vi "Modbus_FSM_Polarization_Control.vi"() -> ()   [LabVIEW 2021]
uses:
  <vilib>/Plasmionique/MB Master/MB_ADU/MB_ADU.lvclass/MB_ADU.ctl
  <vilib>/Plasmionique/MB Master/MB_ADU/Read TX Data.vi
  <vilib>/Plasmionique/MB Master/MB_ADU/Read RX Data.vi
  <vilib>/Plasmionique/MB Master/MB_ADU/Read RX Timestamp.vi
  <vilib>/Plasmionique/MB Master/MB_Master_Serial/MB_Master_Serial.lvclass
  C:/Program Files/National Instruments/LabVIEW 2021/vi.lib/Plasmionique/MB Master/MB_Master/MB_Master.lvclass
  <vilib>/Plasmionique/MB Master/MB_ADU/MB_ADU.lvclass
  <vilib>/Plasmionique/MB Master/MB_Master/MB_Master.lvclass
  <vilib>/Plasmionique/MB Master/MB Master.lvlib
panel:
  out "Full Excitation Scan?":bool=TRUE
  out "Current Excitation HWP Segments":u8=230
  out "Initial Excitation QWP Segments":u8
  out "Current Excitation\nQWP angle":sgl
  in  "Event Registration Refnum":refnum<event-registration>
  in  "stop":bool
  in  "Scan Angle\nExcitation QWP":dbl=45.0
  in  "Excitation Full Scan":bool
  in  "Excitation  QWP Angle":dbl(slide)=1.0 min=0.0 max=180.0 step=0.001 scale=0.0..180.0
  out "Reset Modbus?":bool=TRUE
  in  "Modbus Address":refnum<visa-resource-name>="COM21"
  in  "Collection QWP Angle":dbl(slide)=1.0 min=0.0 max=180.0 step=0.001 scale=0.0..180.0
  in  "Scan Angle \nCollection QWP":dbl=45.0
  in  "Excitation  HWP Angle":dbl(slide)=1.0 min=0.0 max=180.0 step=0.001 scale=0.0..180.0
  in  "Scan Angle \nExcitation HWP":dbl=45.0
  in  "Collection HWP Angle":dbl(slide)=1.0 min=0.0 max=180.0 step=0.1 scale=0.0..180.0
  in  "Scan Angle\nCollection HWP":dbl=45.0
  out "Def Pos CH3":u16[](array[numeric])
  out "Def Pos CH2":u16[](array[numeric])
  out "Def Pos CH1":u16[](array[numeric])
  out "Def Pos CH0":u16[](array[numeric])
  in  "Direction Exc QWP":bool
  in  "Direction Exc HWP":bool
  in  "Direction QWP":bool
  in  "Direction HWP":bool
  out "CH1 Steps/deg":u16=400
  out "CH0 Steps/deg":u16=400
  out "Current Collection HWP Segments":u8
  out "Initial Collection HWP Segments":u8=230
  out "CH2 Steps/deg":u16=400
  out "CH3 Steps/deg":u16=400
  out "Current Collection QWP Segment":u8
  out "Initial Collection QWP Segments":u8=230
  out "Current Collection \nHWP angle":sgl
  out "Current Collection\nQWP angle":sgl
  out "Full Collection Scan?":bool=TRUE
  out "Current Excitation QWP Segments":u8
  out "Initial Excitation HWP Segments":u8=230
  out "Current Excitation\nHWP angle":sgl
  out "Def Pos CH0 Ind":bool=TRUE
  out "Def Pos CH1 Ind":bool=TRUE
  out "Def Pos CH2 Ind":bool=TRUE
  out "Def Pos CH3 Ind":bool=TRUE
  out "Power Dependence?":bool=TRUE
  out "Last RX":string
  out "Last TX":string
  out "Last RX Time":string
  out "dt (ms)":u32=4
  out "Open?":bool
  out "Last Error Time":string
  out "Last Error Status":errorcluster
  in  "Reset Motor":bool
  in  "Excitation QWP":bool
  in  "Excitation HWP":bool
  in  "Collection QWP":bool
  in  "Collection HWP":bool
  in  "Scan Collection polarization":bool
  in  "Absolute Move CH0":bool=TRUE caption="Move to Default"
  in  "Absolute Move CH1":bool=TRUE
  in  "Absolute Move CH2":bool=TRUE
  in  "Absolute Move CH3":bool=TRUE
  in  "Set CH0 Default Position":bool=TRUE caption="Set Default"
  in  "Set CH1 Default Position":bool=TRUE
  in  "Set CH2 Default Position":bool=TRUE
  in  "Set CH3 Default Position":bool=TRUE
  in  "Scan Excitation LP":bool
  in  "Scan Collection LP":bool
  # "Rotation"
  # "Scan"
  # "Direction"
  # "Rotate"
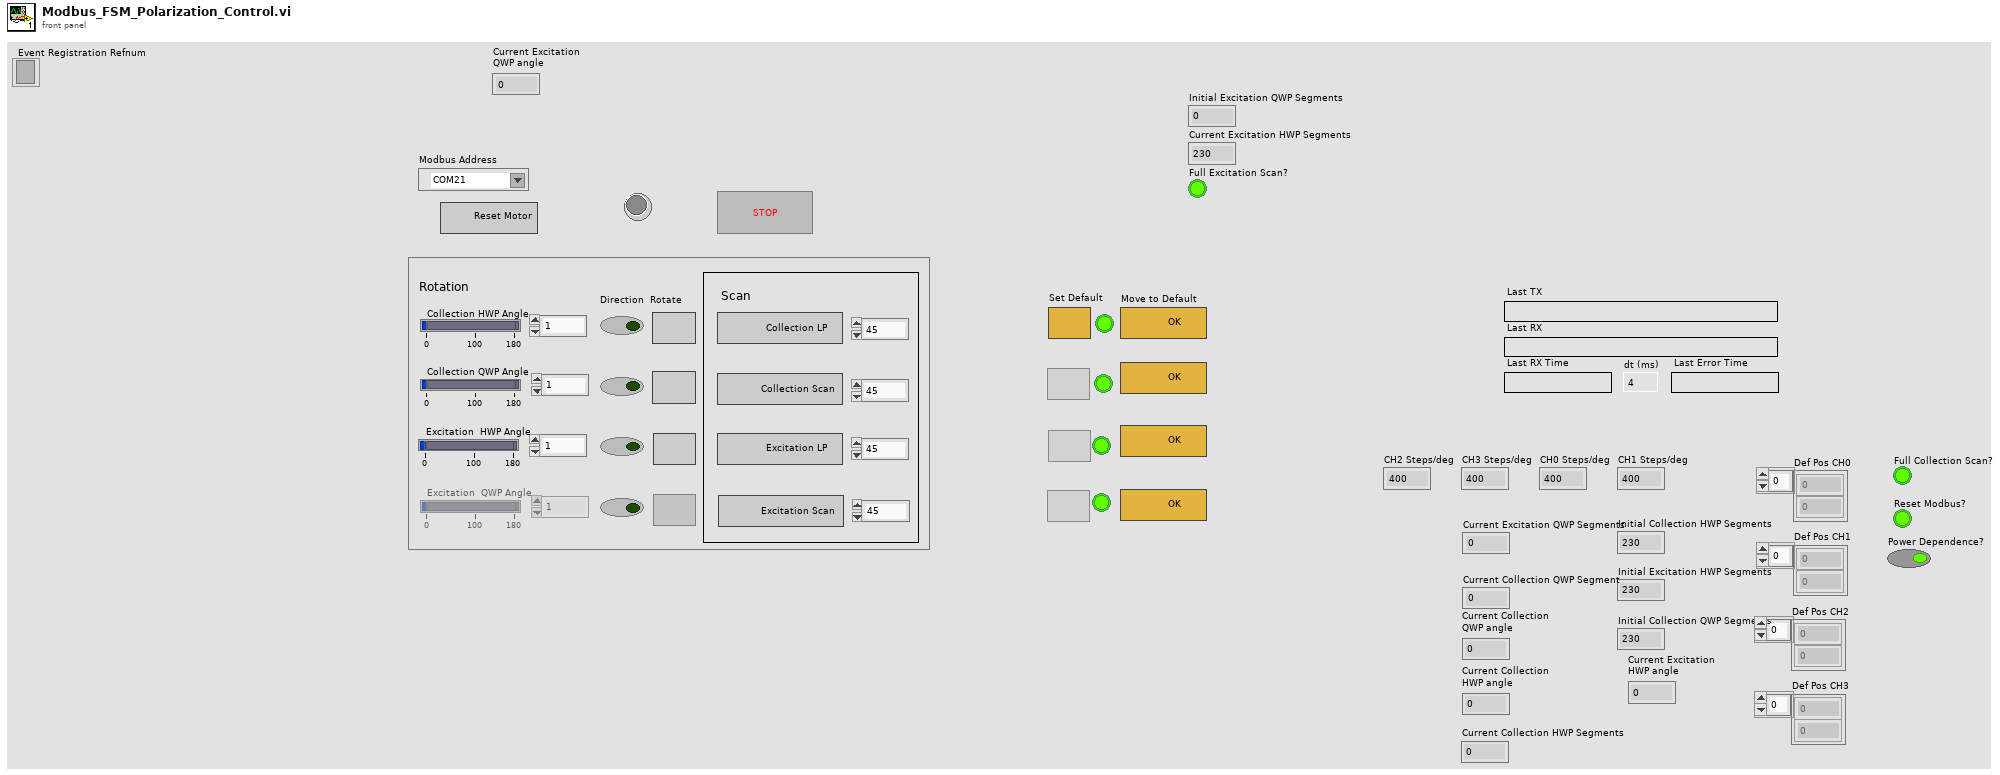
[diagram p1: front panel]
types:
  T1 = cluster{"baud rate (bps)":u32, "stop bits":u16, "parity":u16, "flow control":u16, "timeout":u32, "retries":i32}
  T2 = enum8{"Enabled", "Disabled", "Disabled and Grayed Out"}
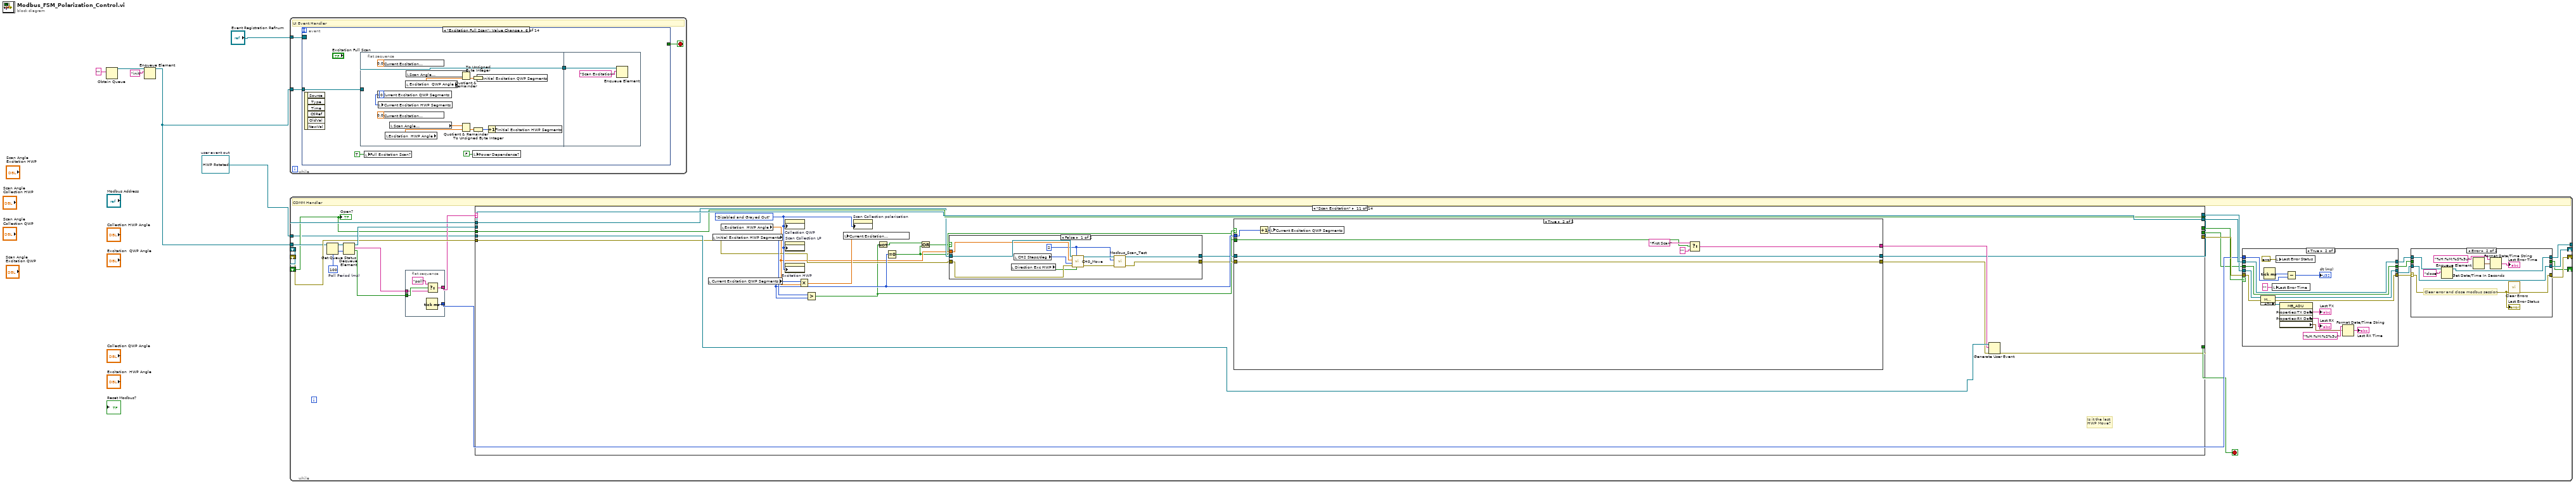
[diagram p0: block diagram]
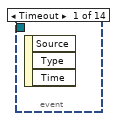
[diagram p2: hidden frame]
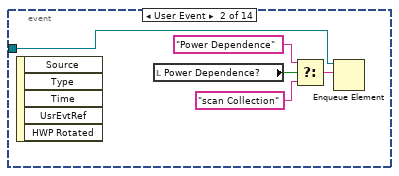
[diagram p3: hidden frame]
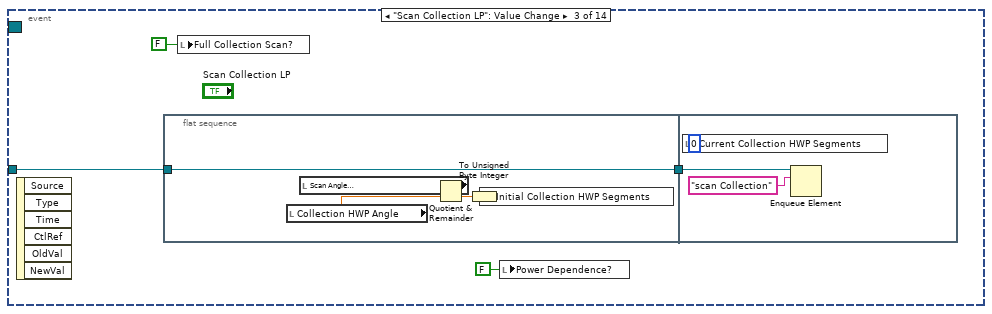
[diagram p4: hidden frame]
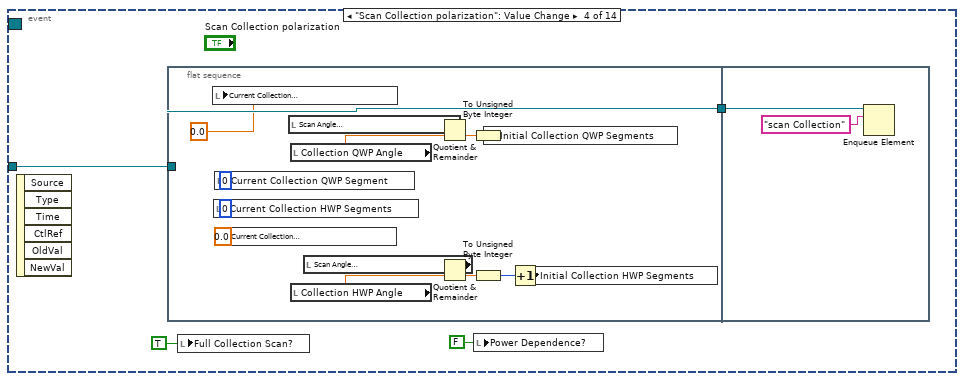
[diagram p5: hidden frame]
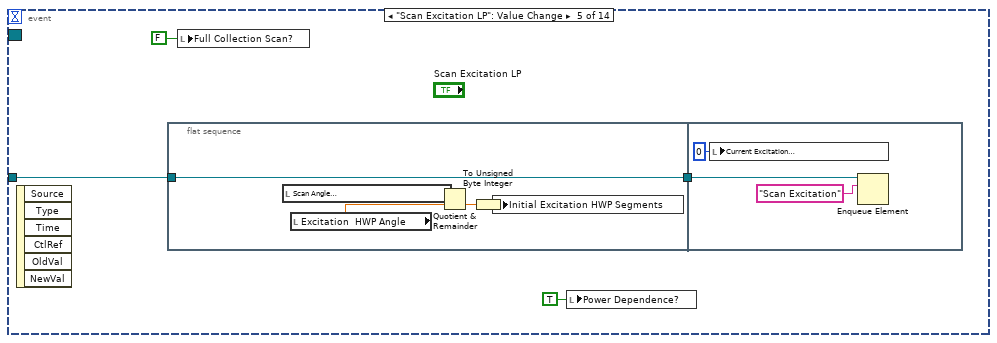
[diagram p6: hidden frame]
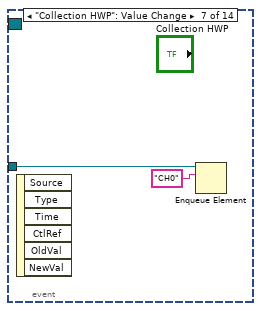
[diagram p7: hidden frame]
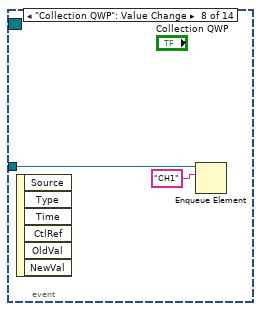
[diagram p8: hidden frame]
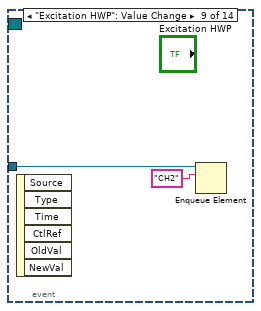
[diagram p9: hidden frame]
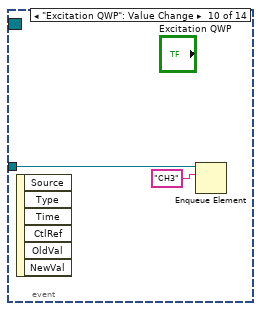
[diagram p10: hidden frame]
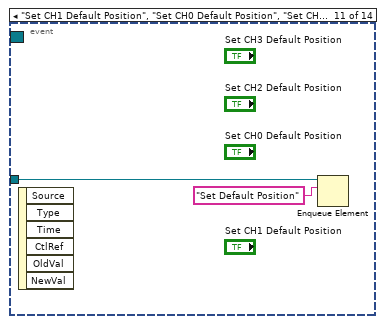
[diagram p11: hidden frame]
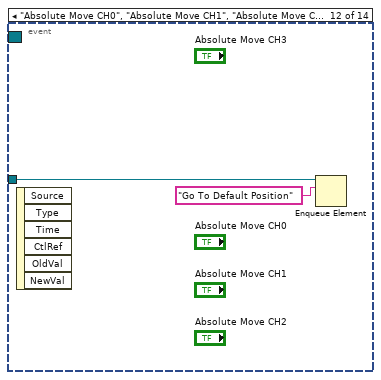
[diagram p12: hidden frame]
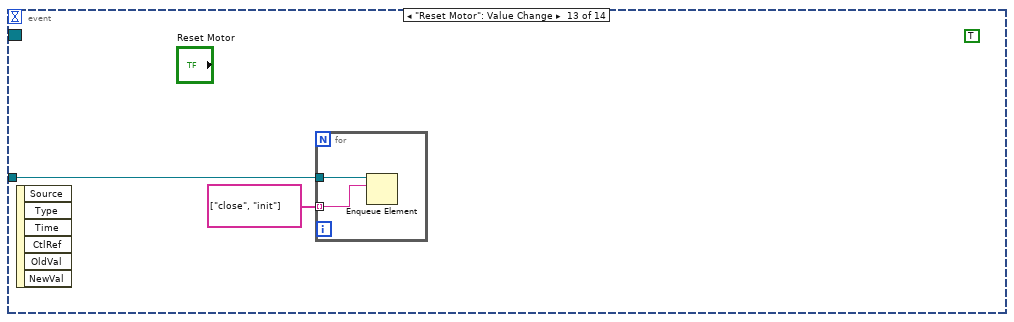
[diagram p13: hidden frame]
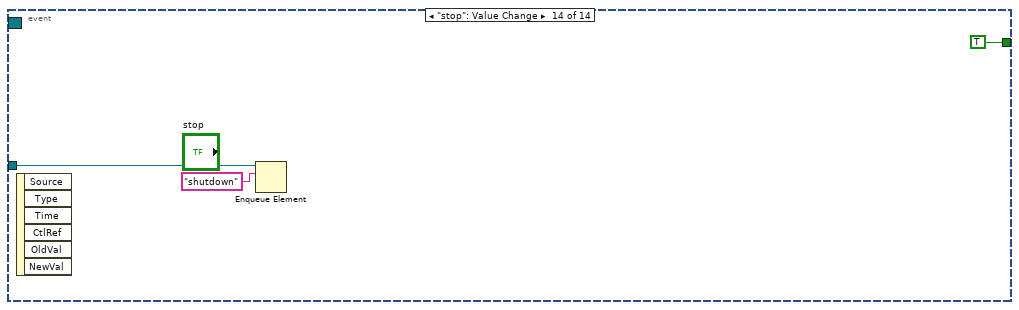
[diagram p14: hidden frame]
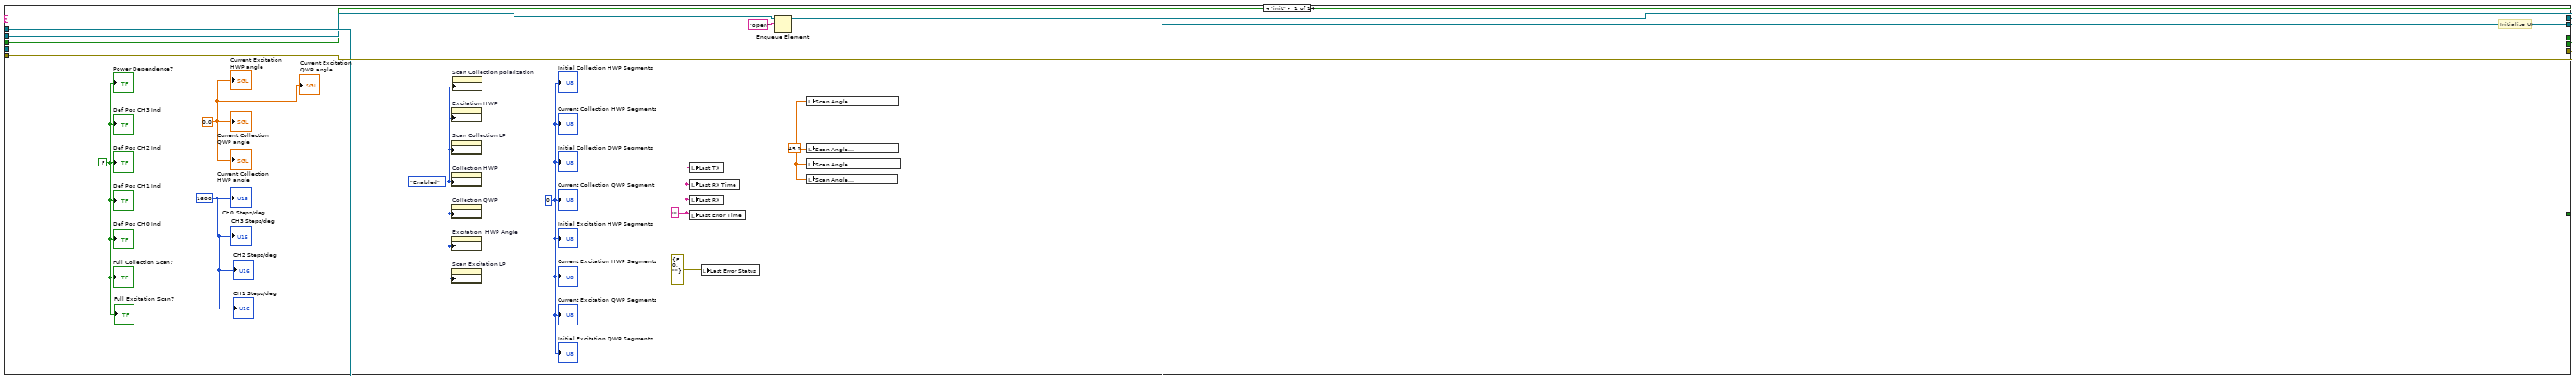
[diagram p17: hidden frame]
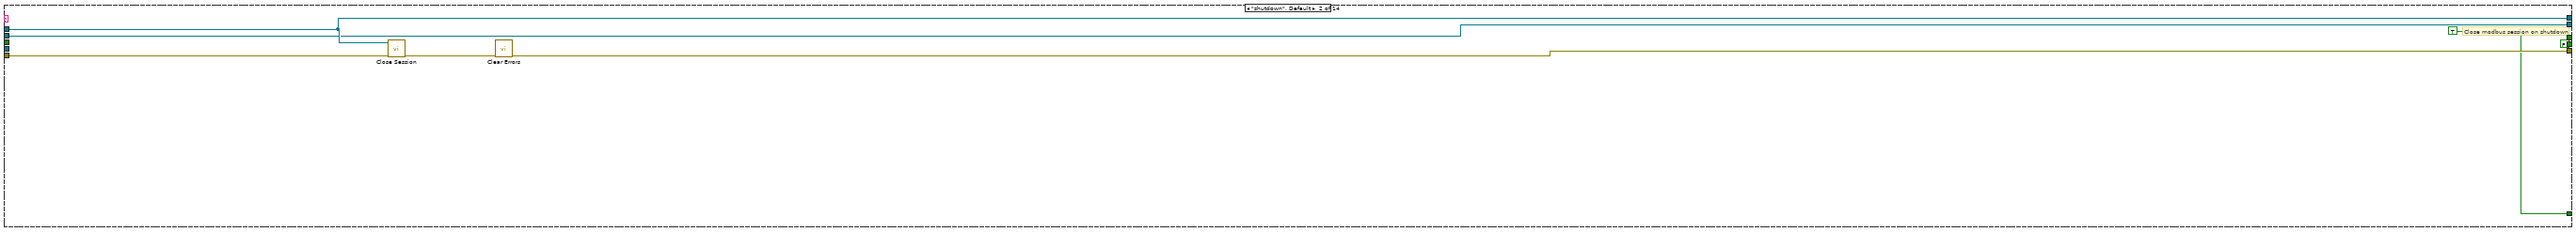
[diagram p18: hidden frame]
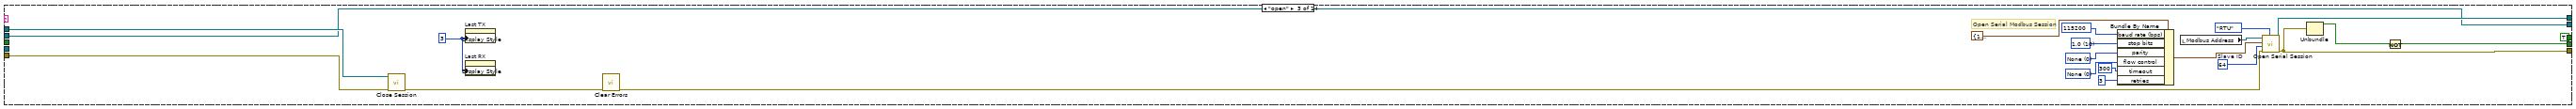
[diagram p19: hidden frame]
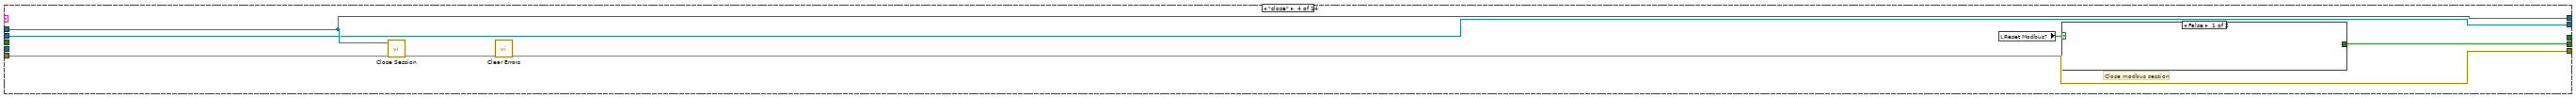
[diagram p20: hidden frame]
diagram:
  w2 = refnum<user-event> refnum  # user event out
  n1 = Obtain Queue(element data type="") -> (queue out=w6:refnum<queue>)  [unwired: 4 in, 2 out]
  n2 = Enqueue Element(queue=w6, element="init") -> (queue out=w3:refnum<queue>)  [unwired: 2 in, 2 out]
  n3 = while {
    tunnel: w3 -> [w9]
    tunnel: "Event Registration Refnum" -> [w7]
    stop <- w8 stop-if-true
    # "UI Event Handler"
    n4 = event shown="[5] \"Excitation Full Scan\": Value Change" {
      selector: w7 -> [_ _ _ _ _ _ _ _ _ _ _ _ _ _]
      dyn-events: _ -> [_ _ _ _ _ _ _ _ _ _ _ _ _ _]
      timeout: _ -> [_ _ _ _ _ _ _ _ _ _ _ _ _ _]
      tunnel: w9 -> [_ w14 w18 w30 w50 w62 w79 w81 w83 w85 w86 w88 w91 w94]
      tunnel: [_ _ _ _ _ _ _ _ _ _ _ _ _ TRUE] -> w8
      event Timeout {
        n5 = event-data() -> ()  [unwired: 1 in, 3 out]
      }
      event User Event {
        n6 = event-data() -> ()  [unwired: 1 in, 5 out]
        n7 = local read "Power Dependence?"() -> (w13:bool)
        n8 = Select(t="Power Dependence" ("element"), s=w13, f="scan Collection" ("element")) -> (s? t:f=w12:string)
        n9 = Enqueue Element(queue=w14, element=w12) -> ()  [unwired: 2 in, 3 out]
      }
      event "Scan Collection LP": Value Change {
        n10 = event-data() -> ()  [unwired: 1 in, 6 out]
        n11 = flat-sequence {
          tunnel: w18 -> [w23]
          tunnel: [w23] -> w17
          tunnel: w17 -> [w25]
          frame #0 {
            n12 = local read "Collection HWP Angle"() -> (w22:dbl)
            n13 = local read "Scan Angle\nCollection HWP"() -> (w19:dbl)
            n14 = Quotient & Remainder(x=w19, y=w22) -> (floor(x/y)=w21:dbl)  [unwired: 1 out]
            n15 = To Unsigned Byte Integer(number=w21) -> (unsigned 8bit integer=w20:u8)
            n16 = local write "Initial Collection HWP Segments"(w20) -> ()
          }
          frame #1 {
            n17 = local write "Current Collection HWP Segments"(u8 0 ("Current HWP Segmen")) -> ()
            n18 = Enqueue Element(queue=w25, element="scan Collection") -> ()  [unwired: 2 in, 3 out]
          }
        }
        n19 = local write "Full Collection Scan?"(FALSE ("Full Collection Scan?")) -> ()
        n20 = local write "Power Dependence?"(FALSE ("Power Dependence?")) -> ()
      }
      event "Scan Collection polarization": Value Change {
        n21 = event-data() -> ()  [unwired: 1 in, 6 out]
        n22 = flat-sequence {
          tunnel: w30 -> [w44]
          tunnel: [w44] -> w29
          tunnel: w29 -> [w45]
          frame #0 {
            n23 = local write "Current Collection \nHWP angle"(sgl 0.0 ("Current HWP angle")) -> ()
            n24 = local write "Current Collection HWP Segments"(u8 0 ("Current HWP Segmen")) -> ()
            n25 = local write "Current Collection QWP Segment"(u8 0 ("Current QWP Segment")) -> ()
            n26 = local write "Current Collection\nQWP angle"(sgl 0.0 ("Current QWP angle")) -> ()
            n27 = local read "Scan Angle \nCollection QWP"() -> (w40:dbl)
            n28 = local read "Collection QWP Angle"() -> (w42:dbl)
            n29 = local read "Collection HWP Angle"() -> (w43:dbl)
            n30 = local read "Scan Angle\nCollection HWP"() -> (w41:dbl)
            n31 = Quotient & Remainder(x=w40, y=w42) -> (floor(x/y)=w38:dbl)  [unwired: 1 out]
            n32 = Quotient & Remainder(x=w41, y=w43) -> (floor(x/y)=w39:dbl)  [unwired: 1 out]
            n33 = To Unsigned Byte Integer(number=w38) -> (unsigned 8bit integer=w31:u8)
            n34 = To Unsigned Byte Integer(number=w39) -> (unsigned 8bit integer=w33:u8)
            n35 = local write "Initial Collection QWP Segments"(w31) -> ()
            n36 = Increment(x=w33) -> (x+1=w32:u8)
            n37 = local write "Initial Collection HWP Segments"(w32) -> ()
          }
          frame #1 {
            n38 = Enqueue Element(queue=w45, element="scan Collection") -> ()  [unwired: 2 in, 3 out]
          }
        }
        n39 = local write "Full Collection Scan?"(TRUE ("Full Collection Scan?")) -> ()
        n40 = local write "Power Dependence?"(FALSE ("Power Dependence?")) -> ()
      }
      event "Scan Excitation LP": Value Change {
        n41 = event-data() -> ()  [unwired: 1 in, 6 out]
        n42 = flat-sequence {
          tunnel: w50 -> [w55]
          tunnel: [w55] -> w49
          tunnel: w49 -> [w57]
          frame #0 {
            n43 = local read "Scan Angle \nExcitation HWP"() -> (w51:dbl)
            n44 = local read "Excitation  HWP Angle"() -> (w54:dbl)
            n45 = Quotient & Remainder(x=w51, y=w54) -> (floor(x/y)=w53:dbl)  [unwired: 1 out]
            n46 = To Unsigned Byte Integer(number=w53) -> (unsigned 8bit integer=w52:u8)
            n47 = local write "Initial Excitation HWP Segments"(w52) -> ()
          }
          frame #1 {
            n48 = local write "Current Excitation\nHWP angle"(u8 0 ("Current HWP Segmen")) -> ()
            n49 = Enqueue Element(queue=w57, element="Scan Excitation") -> ()  [unwired: 2 in, 3 out]
          }
        }
        n50 = local write "Full Collection Scan?"(FALSE ("Full Collection Scan?")) -> ()
        n51 = local write "Power Dependence?"(TRUE ("Power Dependence?")) -> ()
      }
      event "Excitation Full Scan": Value Change {
        n52 = event-data() -> ()  [unwired: 1 in, 6 out]
        n53 = flat-sequence {
          tunnel: w62 -> [w75]
          tunnel: [w75] -> w61
          tunnel: w61 -> [w76]
          frame #0 {
            w63 = u8 0 ("Current QWP Segment")
            n54 = local write "Current Excitation QWP Segments"(w63) -> ()
            n55 = local write "Current Excitation\nHWP angle"(sgl 0.0 ("Current HWP angle")) -> ()
            n56 = local write "Current Excitation HWP Segments"(w63) -> ()
            n57 = local write "Current Excitation\nQWP angle"(sgl 0.0 ("Current QWP angle")) -> ()
            n58 = local read "Excitation  HWP Angle"() -> (w74:dbl)
            n59 = local read "Scan Angle \nExcitation HWP"() -> (w72:dbl)
            n60 = local read "Excitation  QWP Angle"() -> (w73:dbl)
            n61 = local read "Scan Angle\nExcitation QWP"() -> (w71:dbl)
            n62 = Quotient & Remainder(x=w71, y=w73) -> (floor(x/y)=w69:dbl)  [unwired: 1 out]
            n63 = Quotient & Remainder(x=w72, y=w74) -> (floor(x/y)=w70:dbl)  [unwired: 1 out]
            n64 = To Unsigned Byte Integer(number=w69) -> (unsigned 8bit integer=w64:u8)
            n65 = To Unsigned Byte Integer(number=w70) -> (unsigned 8bit integer=w66:u8)
            n66 = local write "Initial Excitation QWP Segments"(w64) -> ()
            n67 = Increment(x=w66) -> (x+1=w65:u8)
            n68 = local write "Initial Excitation HWP Segments"(w65) -> ()
          }
          frame #1 {
            n69 = Enqueue Element(queue=w76, element="Scan Excitation") -> ()  [unwired: 2 in, 3 out]
          }
        }
        n70 = local write "Full Excitation Scan?"(TRUE ("Full Collection Scan?")) -> ()
        n71 = local write "Power Dependence?"(FALSE ("Power Dependence?")) -> ()
      }
      event "Collection HWP": Value Change {
        n72 = event-data() -> ()  [unwired: 1 in, 6 out]
        n73 = Enqueue Element(queue=w79, element="CH0") -> ()  [unwired: 2 in, 3 out]
      }
      event "Collection QWP": Value Change {
        n74 = event-data() -> ()  [unwired: 1 in, 6 out]
        n75 = Enqueue Element(queue=w81, element="CH1") -> ()  [unwired: 2 in, 3 out]
      }
      event "Excitation HWP": Value Change {
        n76 = event-data() -> ()  [unwired: 1 in, 6 out]
        n77 = Enqueue Element(queue=w83, element="CH2") -> ()  [unwired: 2 in, 3 out]
      }
      event "Excitation QWP": Value Change {
        n78 = event-data() -> ()  [unwired: 1 in, 6 out]
        n79 = Enqueue Element(queue=w85, element="CH3") -> ()  [unwired: 2 in, 3 out]
      }
      event "Set CH1 Default Position", "Set CH0 Default Position", "Set CH2 Default Position", "Set CH3 Default Position": Value Change {
        n80 = event-data() -> ()  [unwired: 1 in, 6 out]
        n81 = Enqueue Element(queue=w86, element="Set Default Position") -> ()  [unwired: 2 in, 3 out]
      }
      event "Absolute Move CH0", "Absolute Move CH1", "Absolute Move CH2", "Absolute Move CH3": Value Change {
        n82 = event-data() -> ()  [unwired: 1 in, 6 out]
        n83 = Enqueue Element(queue=w88, element="Go To Default Position") -> ()  [unwired: 2 in, 3 out]
      }
      event "Reset Motor": Value Change {
        (unwired) TRUE
        n84 = event-data() -> ()  [unwired: 1 in, 6 out]
        n85 = for {
          tunnel: w91 -> [w93]
          tunnel: string[] ["close", "init"] ("element") -> [w92] mode=indexing
          n86 = Enqueue Element(queue=w93, element=w92) -> ()  [unwired: 2 in, 3 out]
        }
      }
      event "stop": Value Change {
        n87 = event-data() -> ()  [unwired: 1 in, 6 out]
        n88 = Enqueue Element(queue=w94, element="shutdown") -> ()  [unwired: 2 in, 3 out]
      }
    }
  }
  n89 = while {
    tunnel: w3 -> [w108]
    shift-right: [w113] -> _
    shift-left: _ -> [w122]
    shift-right: [w118] -> _
    shift-left: _ -> [w119]
    tunnel: [w106] -> _
    shift-right: [w100] -> _
    shift-left: _ -> [w103]
    tunnel: w2 -> [w97]
    stop <- w101 stop-if-true
    w120 = 100  # Poll Period (ms)
    # "COMM Handler"
    n90 = Get Queue Status(queue=w108) -> (queue out=w107:refnum<queue>)  [unwired: 2 in, 7 out]
    n91 = Dequeue Element(queue=w107, timeout in ms (-1)=w120) -> (queue out=w121:refnum<queue>, element=w116:string, timed out?=w117:bool)  [unwired: 1 in, 1 out]
    n92 = flat-sequence {
      tunnel: [w140] -> w104
      tunnel: w117 -> [w139]
      tunnel: w116 -> [w138]
      tunnel: [w136] -> w115
      frame #0 {
        n93 = Tick Count (ms)() -> (millisecond timer value=w140:u32)
        n94 = Select(t="poll", s=w139, f=w138) -> (s? t:f=w136:string)
      }
    }
    n95 = case shown="\"Scan Excitation\"" w115 {
      tunnel: [w172 w179 w204 w208 w216 w218 w240 w256 w272 w297 w390 w483 w518 w570] -> w105
      tunnel: w122 -> [w172 w179 w201 w208 w216 w220 w239 w255 w271 w292 w385 w479 w520 w577]
      tunnel: [w174 w180 w203 w209 w217 w223 w241 w257 w273 w303 w396 w489 w519 w573] -> w112
      tunnel: w119 -> [w174 w182 w200 w211 w217 w225 w242 w258 w274 w294 w387 w481 w527 w578]
      tunnel: [w169 FALSE ("EXIT") w197 w205 w214 w219 w238 w254 w270 w299 w392 w485 w517 w569] -> w99
      tunnel: w121 -> [w171 w178 w191 w206 w215 w227 w243 w259 w275 w302 w395 w488 w525 w572]
      tunnel: [w170 w178 w191 w206 w215 w227 w243 w259 w275 w302 w395 w488 w525 w572] -> w109
      tunnel: w97 -> [_ _ _ _ _ _ _ _ _ w305 w398 w491 _ _]
      tunnel: w103 -> [w169 _ _ _ w214 w219 w238 w254 w270 w299 w392 w485 w517 w569]
      tunnel: [_ _ TRUE _ _ w219 w238 w254 w270 w299 w392 w485 w517 w569] -> w102
      tunnel: [_ TRUE _ _ _ _ _ _ _ _ _ _ _ _] -> w101
      frame "init" {
        w162 = FALSE ("Def Pos CH2 Ind")
        w163 = 45.0 ("Scan Angle \nHWP")
        w165 = sgl 0.0 ("Current HWP angle")
        w167 = T2."Enabled" ("Disabled")
        w164 = 0 ("floor(x/y)")
        w166 = u16 1600 ("Etalon Steps/deg")
        w173 = "" ("Last Error Time")
        # "Initialize UI"
        n96 = property on="Excitation HWP" class="Bool"("DisabledEnum"=w167) -> ()  [unwired: 2 in, 2 out]
        n97 = property on="Scan Collection LP" class="Bool"("DisabledEnum"=w167) -> ()  [unwired: 2 in, 2 out]
        n98 = property on="Collection HWP" class="Bool"("DisabledEnum"=w167) -> ()  [unwired: 2 in, 2 out]
        n99 = property on="Collection QWP" class="Bool"("DisabledEnum"=w167) -> ()  [unwired: 2 in, 2 out]
        n100 = property on="Excitation  HWP Angle" class="Slide (strict)"("DisabledEnum"=w167) -> ()  [unwired: 2 in, 2 out]
        n101 = property on="Scan Excitation LP" class="Bool"("DisabledEnum"=w167) -> ()  [unwired: 2 in, 2 out]
        n102 = property on="Scan Collection polarization" class="Bool"("DisabledEnum"=w167) -> ()  [unwired: 2 in, 2 out]
        n103 = local write "Last TX"(w173) -> ()
        n104 = local write "Last RX Time"(w173) -> ()
        n105 = local write "Last RX"(w173) -> ()
        n106 = local write "Last Error Time"(w173) -> ()
        n107 = local write "Last Error Status"(errorcluster {"status"=FALSE, "code"=0, "source"=""} ("Last Error Status")) -> ()
        n108 = Enqueue Element(queue=w171, element="open") -> (queue out=w170:refnum<queue>)  [unwired: 2 in, 2 out]
        n109 = local write "Scan Angle\nCollection HWP"(w163) -> ()
        n110 = local write "Scan Angle \nExcitation HWP"(w163) -> ()
        n111 = local write "Scan Angle \nCollection QWP"(w163) -> ()
        n112 = local write "Scan Angle\nExcitation QWP"(w163) -> ()
        "CH1 Steps/deg" <- w166
        "CH0 Steps/deg" <- w166
        "Current Collection HWP Segments" <- w164
        "Initial Collection HWP Segments" <- w164
        "CH2 Steps/deg" <- w166
        "CH3 Steps/deg" <- w166
        "Current Collection QWP Segment" <- w164
        "Initial Collection QWP Segments" <- w164
        "Current Collection \nHWP angle" <- w165
        "Current Collection\nQWP angle" <- w165
        "Full Collection Scan?" <- w162
        "Current Excitation QWP Segments" <- w164
        "Initial Excitation HWP Segments" <- w164
        "Current Excitation\nHWP angle" <- w165
        "Def Pos CH0 Ind" <- w162
        "Def Pos CH1 Ind" <- w162
        "Def Pos CH2 Ind" <- w162
        "Def Pos CH3 Ind" <- w162
        "Power Dependence?" <- w162
        "Current Excitation\nQWP angle" <- w165
        "Initial Excitation QWP Segments" <- w164
        "Current Excitation HWP Segments" <- w164
        "Full Excitation Scan?" <- w162
      }
      frame "shutdown", Default {
        # "Close modbus session on shutdown"
        n113 = call-dynamic "Close Session.vi"("error in (no error)"=w182, "MB session in"=w179) -> ("error out"=w181:errorcluster)  [unwired: 9 in]
        n114 = call <vilib>:"Clear Errors.vi"("error in (no error)"=w181) -> ("error out"=w180:errorcluster)  [unwired: 5 in, 1 out]
      }
      frame "open" {
        w185 = u32 115200 items=["9600"=9600, "19200"=19200, "38400"=38400, "57600"=57600, "115200"=115200, "460800"=460800, "921600"=921600] ("Baud Rate (bps)")
        w186 = u16 10 items=["1.0"=10, "1.5"=15, "2.0"=20] ("Stop Bits")
        w187 = u16 0 items=["None", "Odd", "Even", "Mark", "Space"] ("Parity")
        w188 = u16 0 items=["None", "XON/XOFF", "RTS/CTS", "XON/XOFF & RTS/CTS", "DTR/DSR", "XON/XOFF & DTR/DSR"] ("Flow Control")
        w192 = u8 64  # Slave ID
        w195 = u32 3 ("Display Style")
        # "Open Serial Modbus Session"
        n115 = call-dynamic "Close Session.vi"("error in (no error)"=w200, "MB session in"=w201) -> ("error out"=w202:errorcluster)  [unwired: 9 in]
        n116 = property on="Last TX" class="Str"("Display Style"=w195) -> ()  [unwired: 2 in, 2 out]
        n117 = property on="Last RX" class="Str"("Display Style"=w195) -> ()  [unwired: 2 in, 2 out]
        n118 = call <vilib>:"Clear Errors.vi"("error in (no error)"=w202) -> ("error out"=w199:errorcluster)  [unwired: 5 in, 1 out]
        n119 = Bundle By Name(cluster=T1 {"baud rate (bps)"=19200, "stop bits"=10, "parity"=0, "flow control"=0, "timeout"=1000, "retries"=1} ("Serial Config"), "baud rate (bps)"=w185, "stop bits"=w186, "parity"=w187, "flow control"=w188, "timeout"=u32 300 ("Timeout (ms)"), "retries"=3 ("Retries")) -> (w183:T1)
        n120 = local read "Modbus Address"() -> (w194:refnum<visa-resource-name>)
        n121 = call <vilib>:"Open Serial Session.vi"("Mode (RTU)"=enum16{"RTU", "ASCII"}."RTU", "Error in"=w199, "Slave ID"=w192, "Serial Config"=w183, "VISA Resource"=w194) -> ("Error out"=w203:errorcluster, "MB_Serial session"=w204:refnum<class "MB_Master_Serial.lvclass">)  [unwired: 5 in]
        n122 = Unbundle(w203) -> ("status"=w196:bool)  [unwired: 2 out]
        n123 = Not(x=w196) -> (.not. x?=w197:bool)
      }
      frame "close" {
        # "Close modbus session"
        n124 = call-dynamic "Close Session.vi"("error in (no error)"=w211, "MB session in"=w208) -> ("error out"=w210:errorcluster)  [unwired: 9 in]
        n125 = call <vilib>:"Clear Errors.vi"("error in (no error)"=w210) -> ("error out"=w209:errorcluster)  [unwired: 5 in, 1 out]
        n126 = local read "Reset Modbus?"() -> (w207:bool)
        n127 = case shown="False" w207 {
          tunnel: [_ FALSE ("stop")] -> w205
          frame False {
          }
          frame True {
            n128 = local write "Reset Modbus?"(FALSE ("Reset Modbus?")) -> ()
          }
        }
      }
      frame "poll" {
        # "Enqueue commands for polled data"
      }
      frame "CH0" {
        n129 = property on="Collection HWP" class="Bool"(error in=w225, "DisabledEnum"=T2."Disabled and Grayed Out" ("Disabled")) -> (error out=w222:errorcluster)  [unwired: 1 in, 1 out]
        n130 = case shown="True" w219 {
          tunnel: w220 -> [w228 w237]
          tunnel: w222 -> [w229 w236]
          tunnel: [w229 w235] -> w221
          tunnel: [w228 w234] -> w218
          frame False {
          }
          frame True {
            n131 = local read "Collection HWP Angle"() -> (w233:dbl)
            n132 = local read "CH0 Steps/deg"() -> (w232:u16)
            n133 = call "CH0_Move.vi"("Direction"="Direction HWP", "Channel"=u8 0, "error in (no error)"=w236, "CH0 Steps/deg"=w232, "Collection HWP Angle"=w233, "MB_Master in"=w237) -> ("error out"=w235:errorcluster, "MB_Master out"=w234:refnum<class "MB_Master.lvclass">)  [unwired: 4 in]
          }
        }
        n134 = property on="Collection HWP" class="Bool"(error in=w221, "DisabledEnum"=T2."Enabled" ("Disabled")) -> (error out=w223:errorcluster)  [unwired: 1 in, 1 out]
      }
      frame "CH1" {
        n135 = case shown="True" w238 {
          tunnel: w239 -> [w244 w253]
          tunnel: w242 -> [w245 w252]
          tunnel: [w245 w251] -> w241
          tunnel: [w244 w250] -> w240
          frame False {
          }
          frame True {
            n136 = local read "Collection QWP Angle"() -> (w249:dbl)
            n137 = local read "CH1 Steps/deg"() -> (w248:u16)
            n138 = call "CH0_Move.vi"("Direction"="Direction QWP", "Channel"=u8 1, "error in (no error)"=w252, "CH0 Steps/deg"=w248, "Collection HWP Angle"=w249, "MB_Master in"=w253) -> ("error out"=w251:errorcluster, "MB_Master out"=w250:refnum<class "MB_Master.lvclass">)  [unwired: 4 in]
          }
        }
      }
      frame "CH2" {
        n139 = case shown="True" w254 {
          tunnel: w255 -> [w260 w269]
          tunnel: w258 -> [w261 w268]
          tunnel: [w261 w267] -> w257
          tunnel: [w260 w266] -> w256
          frame False {
          }
          frame True {
            n140 = local read "Excitation  HWP Angle"() -> (w265:dbl)
            n141 = local read "CH2 Steps/deg"() -> (w264:u16)
            n142 = call "CH0_Move.vi"("Direction"="Direction Exc HWP", "Channel"=u8 2, "error in (no error)"=w268, "CH0 Steps/deg"=w264, "Collection HWP Angle"=w265, "MB_Master in"=w269) -> ("error out"=w267:errorcluster, "MB_Master out"=w266:refnum<class "MB_Master.lvclass">)  [unwired: 4 in]
          }
        }
      }
      frame "CH3" {
        n143 = case shown="True" w270 {
          tunnel: w271 -> [w276 w285]
          tunnel: w274 -> [w277 w284]
          tunnel: [w277 w283] -> w273
          tunnel: [w276 w282] -> w272
          frame False {
          }
          frame True {
            n144 = local read "Excitation  QWP Angle"() -> (w281:dbl)
            n145 = local read "CH3 Steps/deg"() -> (w280:u16)
            n146 = call "CH0_Move.vi"("Direction"="Direction Exc QWP", "Channel"=u8 3, "error in (no error)"=w284, "CH0 Steps/deg"=w280, "Collection HWP Angle"=w281, "MB_Master in"=w285) -> ("error out"=w283:errorcluster, "MB_Master out"=w282:refnum<class "MB_Master.lvclass">)  [unwired: 4 in]
          }
        }
      }
      frame "scan Collection" {
        w296 = T2."Disabled and Grayed Out" ("Disabled")
        # "Is it the last\nHWP Move?"
        n147 = local read "Current Collection HWP Segments"() -> (w295:u8)
        n148 = local read "Initial Collection HWP Segments"() -> (w300:u8)
        n149 = local read "Collection HWP Angle"() -> (w290:dbl)
        n150 = property on="Collection QWP" class="Bool"("DisabledEnum"=w296) -> ()  [unwired: 2 in, 2 out]
        n151 = property on="Scan Collection LP" class="Bool"("DisabledEnum"=w296) -> ()  [unwired: 2 in, 2 out]
        n152 = property on="Collection HWP" class="Bool"("DisabledEnum"=w296) -> ()  [unwired: 2 in, 2 out]
        n153 = Multiply(x=w295, y=w290) -> (x*y=w301:dbl)
        n154 = Greater?(x=w300, y=w295) -> (0:w287:bool)
        n155 = local write "Current Collection \nHWP angle"(w301) -> ()
        n156 = property on="Scan Collection polarization" class="Bool"("DisabledEnum"=w296) -> ()  [unwired: 2 in, 2 out]
        n157 = Not(x=w287) -> (.not. x?=w286:bool)
        n158 = Equal To 0?(x=w295) -> (x = 0?=w289:bool)
        n159 = Or(x=w286, y=w289) -> (x .or. y?=w288:bool)
        n160 = case shown="False" w288 {
          tunnel: w294 -> [w314 w318]
          tunnel: [w309 w318] -> w293
          tunnel: w292 -> [w315 w317]
          tunnel: [w307 w317] -> w291
          tunnel: w290 -> [w313 _]
          frame False {
            w306 = u8 0 ("Channel")
            n161 = local read "CH0 Steps/deg"() -> (w312:u16)
            n162 = local read "Direction HWP"() -> (w311:bool)
            n163 = call "CH0_Move.vi"("Direction"=w311, "Channel"=w306, "error in (no error)"=w314, "CH0 Steps/deg"=w312, "Collection HWP Angle"=w313, "MB_Master in"=w315) -> ("error out"=w310:errorcluster, "MB_Master out"=w308:refnum<class "MB_Master.lvclass">)  [unwired: 4 in]
            n164 = call "Modbus_Scan_Test.vi"("error in (no error)"=w310, "channel"=w306, "MB_Master in"=w308) -> ("error out"=w309:errorcluster, "MB_Master out"=w307:refnum<class "MB_Master.lvclass">)  [unwired: 7 in]
          }
          frame True {
            n165 = Wait (ms)(milliseconds to wait=u32 1000 ("Count(Ticks)")) -> ()  [unwired: 1 out]
          }
        }
        n166 = case shown="False" w287 {
          tunnel: [w324 w378] -> w304
          tunnel: w289 -> [_ w375]
          tunnel: w293 -> [w322 w373]
          tunnel: w291 -> [w321 w374]
          tunnel: [w320 w373] -> w298
          tunnel: [w319 w374] -> w297
          tunnel: w295 -> [_ w371]
          frame False {
            n167 = local read "Full Collection Scan?"() -> (w323:bool)
            n168 = case shown="False" w323 {
              tunnel: ["Last Move" ("t") w340] -> w324
              tunnel: w322 -> [w326 w336]
              tunnel: w321 -> [w327 w338]
              tunnel: [w326 w334] -> w320
              tunnel: [w327 w337] -> w319
              frame False {
                w325 = T2."Enabled" ("Disabled")
                n169 = property on="Collection HWP" class="Bool"("DisabledEnum"=w325) -> ()  [unwired: 2 in, 2 out]
                n170 = property on="Scan Collection LP" class="Bool"("DisabledEnum"=w325) -> ()  [unwired: 2 in, 2 out]
                n171 = property on="Scan Collection polarization" class="Bool"("DisabledEnum"=w325) -> ()  [unwired: 2 in, 2 out]
                n172 = property on="Collection QWP" class="Bool"("DisabledEnum"=w325) -> ()  [unwired: 2 in, 2 out]
              }
              frame True {
                w342 = u8 0 ("Channel")
                # "Rotate the HWP Back to zero\nMove the QWP"
                # "Is it the last QWP Move?"
                n173 = local read "Current Collection \nHWP angle"() -> (w332:sgl)
                n174 = local read "Collection HWP Angle"() -> (w331:dbl)
                n175 = local read "Direction HWP"() -> (w346:bool)
                n176 = local read "CH0 Steps/deg"() -> (w347:u16)
                n177 = Subtract(x=w332, y=w331) -> (x-y=w330:dbl)
                n178 = Not(x=w346) -> (.not. x?=w345:bool)
                n179 = call "CH0_Move.vi"("Direction"=w345, "Channel"=w342, "error in (no error)"=w336, "CH0 Steps/deg"=w347, "Collection HWP Angle"=w330, "MB_Master in"=w338) -> ("error out"=w344:errorcluster, "MB_Master out"=w343:refnum<class "MB_Master.lvclass">)  [unwired: 4 in]
                n180 = call "Modbus_Scan_Test.vi"("error in (no error)"=w344, "channel"=w342, "MB_Master in"=w343) -> ("error out"=w341:errorcluster, "MB_Master out"=w333:refnum<class "MB_Master.lvclass">)  [unwired: 7 in]
                n181 = local read "Current Collection QWP Segment"() -> (w329:u8)
                n182 = local read "Initial Collection QWP Segments"() -> (w348:u8)
                n183 = flat-sequence {
                  tunnel: w341 -> [w349]
                  tunnel: [w349] -> _
                  tunnel: [w349] -> w335
                  frame #0 {
                    n184 = local write "Current Collection \nHWP angle"(sgl 0.0 ("Current HWP angle")) -> ()
                    n185 = local write "Current Collection HWP Segments"(u8 1 ("Current HWP Segmen")) -> ()
                  }
                }
                n186 = Greater?(x=w348, y=w329) -> (0:w339:bool)
                n187 = case shown="True" w339 {
                  tunnel: w335 -> [w354 w370]
                  tunnel: w333 -> [w353 w369]
                  tunnel: [w354 w367] -> w334
                  tunnel: ["Last Move" ("t") "" ("t")] -> w340
                  tunnel: [w353 w360] -> w337
                  tunnel: w329 -> [_ w358]
                  frame False {
                    w352 = T2."Enabled" ("Disabled")
                    n188 = property on="Collection QWP" class="Bool"("DisabledEnum"=w352) -> ()  [unwired: 2 in, 2 out]
                    n189 = property on="Scan Collection LP" class="Bool"("DisabledEnum"=w352) -> ()  [unwired: 2 in, 2 out]
                    n190 = property on="Collection HWP" class="Bool"("DisabledEnum"=w352) -> ()  [unwired: 2 in, 2 out]
                    n191 = property on="Scan Collection polarization" class="Bool"("DisabledEnum"=w352) -> ()  [unwired: 2 in, 2 out]
                  }
                  frame True {
                    w368 = u8 1 ("Channel")
                    n192 = Increment(x=w358) -> (x+1=w357:u8)
                    n193 = local write "Current Collection QWP Segment"(w357) -> ()
                    n194 = local read "Collection QWP Angle"() -> (w356:dbl)
                    n195 = local read "Collection QWP Angle"() -> (w365:dbl)
                    n196 = local read "CH1 Steps/deg"() -> (w364:u16)
                    n197 = local read "Direction QWP"() -> (w362:bool)
                    n198 = Multiply(x=w357, y=w356) -> (x*y=w359:dbl)
                    n199 = call "CH0_Move.vi"("Direction"=w362, "Channel"=w368, "error in (no error)"=w370, "CH0 Steps/deg"=w364, "Collection HWP Angle"=w365, "MB_Master in"=w369) -> ("error out"=w363:errorcluster, "MB_Master out"=w366:refnum<class "MB_Master.lvclass">)  [unwired: 4 in]
                    n200 = local write "Current Collection\nQWP angle"(w359) -> ()
                    n201 = call "Modbus_Scan_Test.vi"("error in (no error)"=w363, "channel"=w368, "MB_Master in"=w366) -> ("error out"=w367:errorcluster, "MB_Master out"=w360:refnum<class "MB_Master.lvclass">)  [unwired: 7 in]
                  }
                }
              }
            }
          }
          frame True {
            n202 = Increment(x=w371) -> (x+1=w372:u8)
            n203 = local write "Current Collection HWP Segments"(w372) -> ()
            n204 = Select(t="First Scan", s=w375, f="") -> (s? t:f=w378:string)
          }
        }
        n205 = Generate User Event(user event=w305, event data cluster=w304, error in=w298) -> (error out=w303:errorcluster)  [unwired: 1 in, 1 out]
      }
      frame "Scan Excitation" {
        w389 = T2."Disabled and Grayed Out" ("Disabled")
        # "Is it the last\nHWP Move?"
        n206 = local read "Current Excitation QWP Segments"() -> (w388:u8)
        n207 = local read "Initial Excitation HWP Segments"() -> (w393:u8)
        n208 = local read "Excitation  HWP Angle"() -> (w383:dbl)
        n209 = property on="Collection QWP" class="Bool"("DisabledEnum"=w389) -> ()  [unwired: 2 in, 2 out]
        n210 = property on="Scan Collection LP" class="Bool"("DisabledEnum"=w389) -> ()  [unwired: 2 in, 2 out]
        n211 = property on="Excitation HWP" class="Bool"("DisabledEnum"=w389) -> ()  [unwired: 2 in, 2 out]
        n212 = Multiply(x=w388, y=w383) -> (x*y=w394:dbl)
        n213 = Greater?(x=w393, y=w388) -> (0:w380:bool)
        n214 = local write "Current Excitation\nHWP angle"(w394) -> ()
        n215 = property on="Scan Collection polarization" class="Bool"("DisabledEnum"=w389) -> ()  [unwired: 2 in, 2 out]
        n216 = Not(x=w380) -> (.not. x?=w379:bool)
        n217 = Equal To 0?(x=w388) -> (x = 0?=w382:bool)
        n218 = Or(x=w379, y=w382) -> (x .or. y?=w381:bool)
        n219 = case shown="False" w381 {
          tunnel: w387 -> [w407 w411]
          tunnel: [w402 w411] -> w386
          tunnel: w385 -> [w408 w410]
          tunnel: [w400 w410] -> w384
          tunnel: w383 -> [w406 _]
          frame False {
            w399 = u8 2 ("Channel")
            n220 = local read "Direction Exc HWP"() -> (w404:bool)
            n221 = local read "CH2 Steps/deg"() -> (w405:u16)
            n222 = call "CH0_Move.vi"("Direction"=w404, "Channel"=w399, "error in (no error)"=w407, "CH0 Steps/deg"=w405, "Collection HWP Angle"=w406, "MB_Master in"=w408) -> ("error out"=w403:errorcluster, "MB_Master out"=w401:refnum<class "MB_Master.lvclass">)  [unwired: 4 in]
            n223 = call "Modbus_Scan_Test.vi"("error in (no error)"=w403, "channel"=w399, "MB_Master in"=w401) -> ("error out"=w402:errorcluster, "MB_Master out"=w400:refnum<class "MB_Master.lvclass">)  [unwired: 7 in]
          }
          frame True {
            n224 = Wait (ms)(milliseconds to wait=u32 1000 ("Count(Ticks)")) -> ()  [unwired: 1 out]
          }
        }
        n225 = case shown="True" w380 {
          tunnel: [w417 w471] -> w397
          tunnel: w382 -> [_ w468]
          tunnel: w386 -> [w415 w466]
          tunnel: w384 -> [w414 w467]
          tunnel: [w413 w466] -> w391
          tunnel: [w412 w467] -> w390
          tunnel: w388 -> [_ w464]
          frame False {
            n226 = local read "Full Excitation Scan?"() -> (w416:bool)
            n227 = case shown="False" w416 {
              tunnel: ["Last Move" ("t") w433] -> w417
              tunnel: w415 -> [w419 w429]
              tunnel: w414 -> [w420 w431]
              tunnel: [w419 w427] -> w413
              tunnel: [w420 w430] -> w412
              frame False {
                w418 = T2."Enabled" ("Disabled")
                n228 = property on="Collection HWP" class="Bool"("DisabledEnum"=w418) -> ()  [unwired: 2 in, 2 out]
                n229 = property on="Scan Collection LP" class="Bool"("DisabledEnum"=w418) -> ()  [unwired: 2 in, 2 out]
                n230 = property on="Scan Collection polarization" class="Bool"("DisabledEnum"=w418) -> ()  [unwired: 2 in, 2 out]
                n231 = property on="Collection QWP" class="Bool"("DisabledEnum"=w418) -> ()  [unwired: 2 in, 2 out]
              }
              frame True {
                w435 = u8 2 ("Channel")
                # "Rotate the HWP Back to zero\nMove the QWP"
                # "Is it the last QWP Move?"
                n232 = local read "Current Excitation\nHWP angle"() -> (w425:sgl)
                n233 = local read "Excitation  HWP Angle"() -> (w424:dbl)
                n234 = local read "Direction Exc HWP"() -> (w439:bool)
                n235 = local read "CH2 Steps/deg"() -> (w440:u16)
                n236 = Subtract(x=w425, y=w424) -> (x-y=w423:dbl)
                n237 = Not(x=w439) -> (.not. x?=w438:bool)
                n238 = call "CH0_Move.vi"("Direction"=w438, "Channel"=w435, "error in (no error)"=w429, "CH0 Steps/deg"=w440, "Collection HWP Angle"=w423, "MB_Master in"=w431) -> ("error out"=w437:errorcluster, "MB_Master out"=w436:refnum<class "MB_Master.lvclass">)  [unwired: 4 in]
                n239 = call "Modbus_Scan_Test.vi"("error in (no error)"=w437, "channel"=w435, "MB_Master in"=w436) -> ("error out"=w434:errorcluster, "MB_Master out"=w426:refnum<class "MB_Master.lvclass">)  [unwired: 7 in]
                n240 = local read "Current Excitation QWP Segments"() -> (w422:u8)
                n241 = local read "Initial Excitation QWP Segments"() -> (w441:u8)
                n242 = flat-sequence {
                  tunnel: w434 -> [w442]
                  tunnel: [w442] -> _
                  tunnel: [w442] -> w428
                  frame #0 {
                    n243 = local write "Current Excitation\nHWP angle"(sgl 0.0 ("Current HWP angle")) -> ()
                    n244 = local write "Current Excitation HWP Segments"(u8 1 ("Current HWP Segmen")) -> ()
                  }
                }
                n245 = Greater?(x=w441, y=w422) -> (0:w432:bool)
                n246 = case shown="True" w432 {
                  tunnel: w428 -> [w447 w463]
                  tunnel: w426 -> [w446 w462]
                  tunnel: [w447 w460] -> w427
                  tunnel: ["Last Move" ("t") "" ("t")] -> w433
                  tunnel: [w446 w453] -> w430
                  tunnel: w422 -> [_ w451]
                  frame False {
                    w445 = T2."Enabled" ("Disabled")
                    n247 = property on="Collection QWP" class="Bool"("DisabledEnum"=w445) -> ()  [unwired: 2 in, 2 out]
                    n248 = property on="Scan Collection LP" class="Bool"("DisabledEnum"=w445) -> ()  [unwired: 2 in, 2 out]
                    n249 = property on="Collection HWP" class="Bool"("DisabledEnum"=w445) -> ()  [unwired: 2 in, 2 out]
                    n250 = property on="Scan Collection polarization" class="Bool"("DisabledEnum"=w445) -> ()  [unwired: 2 in, 2 out]
                  }
                  frame True {
                    w461 = u8 3 ("Channel")
                    n251 = Increment(x=w451) -> (x+1=w450:u8)
                    n252 = local write "Current Excitation QWP Segments"(w450) -> ()
                    n253 = local read "Excitation  QWP Angle"() -> (w449:dbl)
                    n254 = local read "Excitation  QWP Angle"() -> (w458:dbl)
                    n255 = local read "Direction Exc QWP"() -> (w455:bool)
                    n256 = local read "CH3 Steps/deg"() -> (w457:u16)
                    n257 = Multiply(x=w450, y=w449) -> (x*y=w452:dbl)
                    n258 = call "CH0_Move.vi"("Direction"=w455, "Channel"=w461, "error in (no error)"=w463, "CH0 Steps/deg"=w457, "Collection HWP Angle"=w458, "MB_Master in"=w462) -> ("error out"=w456:errorcluster, "MB_Master out"=w459:refnum<class "MB_Master.lvclass">)  [unwired: 4 in]
                    n259 = local write "Current Excitation\nQWP angle"(w452) -> ()
                    n260 = call "Modbus_Scan_Test.vi"("error in (no error)"=w456, "channel"=w461, "MB_Master in"=w459) -> ("error out"=w460:errorcluster, "MB_Master out"=w453:refnum<class "MB_Master.lvclass">)  [unwired: 7 in]
                  }
                }
              }
            }
          }
          frame True {
            n261 = Increment(x=w464) -> (x+1=w465:u8)
            n262 = local write "Current Excitation QWP Segments"(w465) -> ()
            n263 = Select(t="First Scan", s=w468, f="") -> (s? t:f=w471:string)
          }
        }
        n264 = Generate User Event(user event=w398, event data cluster=w397, error in=w391) -> (error out=w396:errorcluster)  [unwired: 1 in, 1 out]
      }
      frame "Power Dependence" {
        w472 = T2."Disabled and Grayed Out" ("Disabled")
        # "Is it the last\nHWP Move?"
        n265 = local read "Current Excitation QWP Segments"() -> (w482:u8)
        n266 = local read "Initial Excitation HWP Segments"() -> (w486:u8)
        n267 = local read "Excitation  HWP Angle"() -> (w477:dbl)
        n268 = property on="Collection QWP" class="Bool"("DisabledEnum"=w472) -> ()  [unwired: 2 in, 2 out]
        n269 = property on="Scan Collection LP" class="Bool"("DisabledEnum"=w472) -> ()  [unwired: 2 in, 2 out]
        n270 = property on="Excitation  HWP Angle" class="Slide (strict)"("DisabledEnum"=w472) -> ()  [unwired: 2 in, 2 out]
        n271 = property on="Collection HWP" class="Bool"("DisabledEnum"=w472) -> ()  [unwired: 2 in, 2 out]
        n272 = Multiply(x=w482, y=w477) -> (x*y=w487:dbl)
        n273 = Greater?(x=w486, y=w482) -> (0:w474:bool)
        n274 = local write "Current Excitation QWP Segments"(w487) -> ()
        n275 = property on="Scan Collection polarization" class="Bool"("DisabledEnum"=w472) -> ()  [unwired: 2 in, 2 out]
        n276 = property on="Scan Excitation LP" class="Bool"("DisabledEnum"=w472) -> ()  [unwired: 2 in, 2 out]
        n277 = Not(x=w474) -> (.not. x?=w473:bool)
        n278 = Equal To 0?(x=w482) -> (x = 0?=w476:bool)
        n279 = Or(x=w473, y=w476) -> (x .or. y?=w475:bool)
        n280 = case shown="False" w475 {
          tunnel: w481 -> [w500 w504]
          tunnel: [w495 w504] -> w480
          tunnel: w479 -> [w501 w503]
          tunnel: [w493 w503] -> w478
          tunnel: w477 -> [w499 _]
          frame False {
            w492 = u8 2 ("Channel")
            n281 = local read "Direction Exc HWP"() -> (w497:bool)
            n282 = local read "CH2 Steps/deg"() -> (w498:u16)
            n283 = call "CH0_Move.vi"("Direction"=w497, "Channel"=w492, "error in (no error)"=w500, "CH0 Steps/deg"=w498, "Collection HWP Angle"=w499, "MB_Master in"=w501) -> ("error out"=w496:errorcluster, "MB_Master out"=w494:refnum<class "MB_Master.lvclass">)  [unwired: 4 in]
            n284 = call "Modbus_Scan_Test.vi"("error in (no error)"=w496, "channel"=w492, "MB_Master in"=w494) -> ("error out"=w495:errorcluster, "MB_Master out"=w493:refnum<class "MB_Master.lvclass">)  [unwired: 7 in]
          }
          frame True {
            n285 = Wait (ms)(milliseconds to wait=u32 1000 ("Count(Ticks)")) -> ()  [unwired: 1 out]
          }
        }
        n286 = case shown="False" w474 {
          tunnel: ["Last Move" ("t") w516] -> w490
          tunnel: w476 -> [_ w513]
          tunnel: w480 -> [w507 w511]
          tunnel: w478 -> [w506 w512]
          tunnel: [w507 w511] -> w484
          tunnel: [w506 w512] -> w483
          tunnel: w482 -> [_ w509]
          frame False {
            w505 = T2."Enabled" ("Disabled")
            n287 = property on="Excitation  HWP Angle" class="Slide (strict)"("DisabledEnum"=w505) -> ()  [unwired: 2 in, 2 out]
            n288 = property on="Scan Excitation LP" class="Bool"("DisabledEnum"=w505) -> ()  [unwired: 2 in, 2 out]
            n289 = property on="Collection HWP" class="Bool"("DisabledEnum"=w505) -> ()  [unwired: 2 in, 2 out]
            n290 = property on="Scan Collection LP" class="Bool"("DisabledEnum"=w505) -> ()  [unwired: 2 in, 2 out]
            n291 = property on="Scan Collection polarization" class="Bool"("DisabledEnum"=w505) -> ()  [unwired: 2 in, 2 out]
            n292 = property on="Collection QWP" class="Bool"("DisabledEnum"=w505) -> ()  [unwired: 2 in, 2 out]
          }
          frame True {
            n293 = Increment(x=w509) -> (x+1=w510:u8)
            n294 = local write "Current Excitation QWP Segments"(w510) -> ()
            n295 = Select(t="First Scan", s=w513, f="") -> (s? t:f=w516:string)
          }
        }
        n296 = Generate User Event(user event=w491, event data cluster=w490, error in=w484) -> (error out=w489:errorcluster)  [unwired: 1 in, 1 out]
      }
      frame "Go To Default Position" {
        n297 = local read "Absolute Move CH0"() -> (w538:bool)
        n298 = local read "Absolute Move CH1"() -> (w537:bool)
        n299 = local read "Absolute Move CH2"() -> (w536:bool)
        n300 = local read "Absolute Move CH3"() -> (w535:bool)
        n301 = case shown="True" w538 {
          tunnel: [_ "CH0"] -> w534
          frame False {
          }
          frame True {
            n302 = local write "Absolute Move CH0"(FALSE ("Get CH0 Default Position")) -> ()
          }
        }
        n303 = case shown="True" w537 {
          tunnel: [_ "CH1"] -> w533
          frame False {
          }
          frame True {
            n304 = local write "Absolute Move CH1"(FALSE ("Get CH0 Default Position")) -> ()
          }
        }
        n305 = case shown="True" w536 {
          tunnel: [_ "CH2"] -> w532
          frame False {
          }
          frame True {
            n306 = local write "Absolute Move CH2"(FALSE ("Get CH0 Default Position")) -> ()
          }
        }
        n307 = case shown="True" w535 {
          tunnel: [_ "CH3"] -> w531
          frame False {
          }
          frame True {
            n308 = local write "Absolute Move CH3"(FALSE ("Get CH0 Default Position")) -> ()
          }
        }
        n309 = Concatenate Strings(w534, w533, w532, w531) -> (w526:string)
        n310 = case shown="\"CH0\"" w526 {
          tunnel: w527 -> [_ w551 w554 w557 w560]
          tunnel: [errorcluster {"status"=TRUE, "code"=0, "source"="Absolute Position Movement \nAbs Move CH ERROR"} ("error out") w551 w554 w557 w560] -> w521
          tunnel: [_ w550 w553 w555 w559] -> w522
          tunnel: [999 0 ("y") 1 ("x") 2 ("x") 3 ("x")] -> w524
          frame "False", Default {
          }
          frame "CH0" {
            n311 = local read "Def Pos CH0"() -> (w550:u16[])
          }
          frame "CH1" {
            n312 = local read "Def Pos CH1"() -> (w553:u16[])
          }
          frame "CH2" {
            n313 = local read "Def Pos CH0"() -> (w555:u16[])
          }
          frame "CH3" {
            n314 = local read "Def Pos CH3"() -> (w559:u16[])
          }
        }
        n315 = Multiply(x=w524, y=100) -> (x*y=w528:i32)
        n316 = Add(x=10116, y=w528) -> (x+y=w523:i32)
        n317 = case shown="True" w517 {
          tunnel: w520 -> [w540 w546]
          tunnel: w523 -> [_ w545]
          tunnel: w521 -> [w539 w544]
          tunnel: w522 -> [_ w541]
          tunnel: [w540 w543] -> w518
          tunnel: [w539 w542] -> w519
          frame False {
          }
          frame True {
            n318 = call <vilib>:"Write Multiple Registers.vi"("error in (no error)"=w544, "values"=w541, "starting address"=w545, "MB session in"=w546) -> ("error out"=w542:errorcluster, "MB session out"=w543:refnum<class "MB_Master.lvclass">)  [unwired: 6 in]
          }
        }
      }
      frame "Set Default Position" {
        n319 = local read "Set CH0 Default Position"() -> (w591:bool)
        n320 = local read "Set CH1 Default Position"() -> (w590:bool)
        n321 = local read "Set CH2 Default Position"() -> (w589:bool)
        n322 = local read "Set CH3 Default Position"() -> (w588:bool)
        n323 = case shown="True" w591 {
          tunnel: [_ "Get CH0 Default Position"] -> w587
          frame False {
          }
          frame True {
            n324 = local write "Set CH0 Default Position"(FALSE ("Get CH0 Default Position")) -> ()
          }
        }
        n325 = case shown="True" w590 {
          tunnel: [_ "Get CH1 Default Position"] -> w586
          frame False {
          }
          frame True {
            n326 = local write "Set CH1 Default Position"(FALSE ("Get CH0 Default Position")) -> ()
          }
        }
        n327 = case shown="True" w589 {
          tunnel: [_ "Get CH2 Default Position"] -> w585
          frame False {
          }
          frame True {
            n328 = local write "Set CH2 Default Position"(FALSE ("Get CH0 Default Position")) -> ()
          }
        }
        n329 = case shown="True" w588 {
          tunnel: [_ "Get CH3 Default Position"] -> w584
          frame False {
          }
          frame True {
            n330 = local write "Set CH3 Default Position"(FALSE ("Get CH0 Default Position")) -> ()
          }
        }
        n331 = Concatenate Strings(w587, w586, w585, w584) -> (w576:string)
        n332 = case shown="\"False\", Default" w576 {
          tunnel: [999 0 1 2 3] -> w571
          tunnel: w578 -> [_ w619 w621 w623 w625]
          tunnel: [errorcluster {"status"=TRUE, "code"=0, "source"=""} ("error out 2") w619 w621 w623 w625] -> w579
          frame "False", Default {
          }
          frame "Get CH0 Default Position" {
          }
          frame "Get CH1 Default Position" {
          }
          frame "Get CH2 Default Position" {
          }
          frame "Get CH3 Default Position" {
          }
        }
        n333 = Multiply(x=w571, y=100) -> (x*y=w581:i32)
        n334 = Add(x=10102, y=w581) -> (x+y=w580:i32)
        n335 = case shown="True" w569 {
          tunnel: w577 -> [w609 w616]
          tunnel: w580 -> [_ w615]
          tunnel: w579 -> [w608 w613]
          tunnel: [w608 w612] -> w574
          tunnel: [w609 w611] -> w570
          tunnel: [w606 w610] -> w575
          frame False {
            n336 = Build Array(u16 0, u16 0 ("element")) -> (w606:u16[])
          }
          frame True {
            n337 = call <vilib>:"Read Holding Registers.vi"("error in (no error)"=w613, "quantity"=u16 2, "starting address"=w615, "MB session in"=w616) -> ("error out"=w612:errorcluster, "Registers"=w610:u16[], "MB session out"=w611:refnum<class "MB_Master.lvclass">)  [unwired: 5 in]
          }
        }
        n338 = case shown="\"False\", Default" w576 {
          tunnel: w575 -> [_ w595 w598 w601 w604]
          tunnel: w574 -> [w592 w594 w597 w600 w603]
          tunnel: [w592 w594 w597 w600 w603] -> w573
          frame "False", Default {
          }
          frame "Get CH0 Default Position" {
            n339 = local write "Def Pos CH0 Ind"(TRUE ("Def Pos CH0 Ind")) -> ()
            "Def Pos CH0" <- w595
          }
          frame "Get CH1 Default Position" {
            n340 = local write "Def Pos CH1 Ind"(TRUE ("Def Pos CH0 Ind")) -> ()
            "Def Pos CH1" <- w598
          }
          frame "Get CH2 Default Position" {
            n341 = local write "Def Pos CH2 Ind"(TRUE ("Def Pos CH0 Ind")) -> ()
            "Def Pos CH2" <- w601
          }
          frame "Get CH3 Default Position" {
            n342 = local write "Def Pos CH3 Ind"(TRUE ("Def Pos CH0 Ind")) -> ()
            "Def Pos CH3" <- w604
          }
        }
      }
    }
    n343 = case shown="True" w102 {
      tunnel: w105 -> [w144 w148]
      tunnel: [w144 w159] -> w114
      tunnel: w104 -> [_ w153]
      tunnel: w112 -> [w143 w147]
      tunnel: [w143 w146] -> w111
      tunnel: w109 -> [w142 w149]
      tunnel: [w142 w149] -> w110
      tunnel: w99 -> [w141 w145]
      tunnel: [w141 w145] -> w98
      frame False {
      }
      frame True {
        n344 = property class="MB_Master"(reference=w148, error in=w147) -> (reference out=w159:refnum<class "MB_Master.lvclass">, error out=w146:errorcluster, "Properties:ADU"=w160:refnum<class "MB_ADU.lvclass">)
        n345 = Tick Count (ms)() -> (millisecond timer value=w152:u32)
        n346 = local write "Last Error Time"("" ("Last Error Time")) -> ()
        n347 = local write "Last Error Status"(errorcluster {"status"=FALSE, "code"=0, "source"=""} ("Last Error Status")) -> ()
        n348 = property class="MB_ADU"(reference=w160) -> ("Properties:TX Data"=→"Last TX":string, "Properties:RX Data"=→"Last RX":string, "Properties:RX Timestamp"=w150:timestamp)  [unwired: 1 in, 2 out]
        n349 = Subtract(x=w152, y=w153) -> (x-y=→"dt (ms)":u32)
        n350 = Format Date/Time String(time format string (%c)="%H:%M:%S%3u", seconds (now)=w150) -> (date/time string=→"Last RX Time":string)  [unwired: 1 in]
      }
    }
    n351 = case shown="Error" w111 {
      selector: w111 -> [w126 w128]
      tunnel: [w126 w132] -> w118
      tunnel: w110 -> [w125 w130]
      tunnel: [w125 w129] -> w106
      tunnel: w114 -> [w124 w127]
      tunnel: [w124 w127] -> w113
      tunnel: w98 -> [w123 _]
      tunnel: [w123 _] -> w100
      frame No Error {
      }
      frame Error {
        # "Clear error and close modbus session"
        n352 = Enqueue Element(queue=w130, element="close") -> (queue out=w129:refnum<queue>)  [unwired: 2 in, 2 out]
        n353 = Get Date/Time In Seconds() -> (seconds since 1Jan1904=w133:timestamp)
        n354 = Format Date/Time String(time format string (%c)="%H:%M:%S%3u", seconds (now)=w133) -> (date/time string=→"Last Error Time":string)  [unwired: 1 in]
        n355 = call <vilib>:"Clear Errors.vi"("error in (no error)"=w128) -> ("error out"=w132:errorcluster)  [unwired: 5 in, 1 out]
        "Last Error Status" <- w128
      }
    }
    "Open?" <- w103
  }
